vi "Secuencia_Leds.vi"() -> ()   [LabVIEW 2020]
panel:
  out "Array":bool[](array[boolean])
  out "data":bool[](array[boolean])
  out "Numeric":dbl
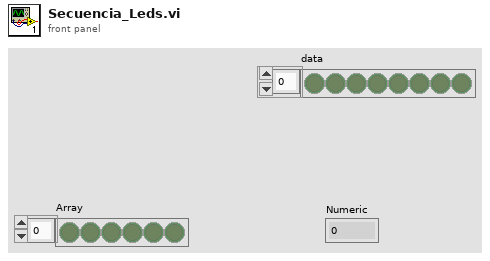
[diagram p1: front panel]
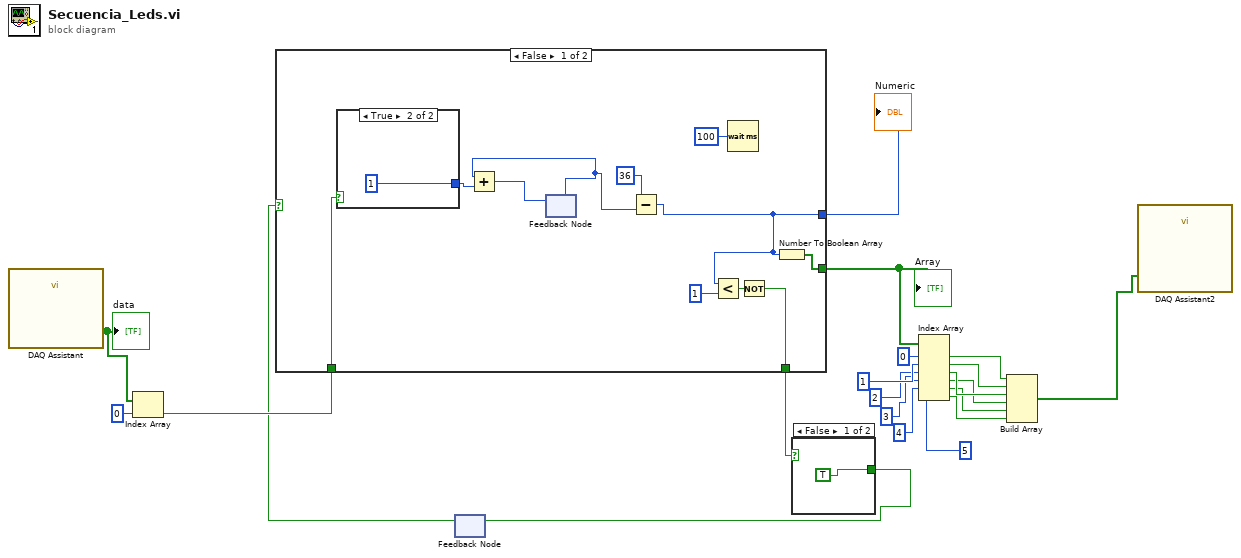
[diagram p0: block diagram]
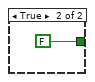
[diagram p2: hidden frame]
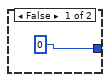
[diagram p3: hidden frame]
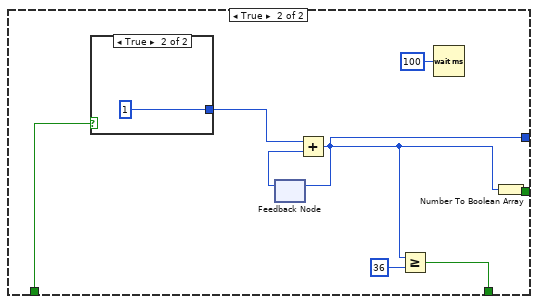
[diagram p4: hidden frame]
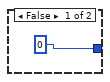
[diagram p5: hidden frame]
diagram:
  n1 = call "DAQ Assistant"() -> ("data"=w21:bool[])  [unwired: 17 in, 2 out]
  "data" <- w21
  n2 = Index Array(array=w21, index=0) -> (element=w19:bool)
  n3 = feedback #1() -> (w2:bool)  [unwired: 1 in]
  n4 = case shown="False" w2 {
    tunnel: [w32 w42] -> w17
    tunnel: w19 -> [w30 w41]
    tunnel: [w25 w37] -> w18
    tunnel: [w23 w35] -> w1
    frame False {
      n5 = case shown="True" w30 {
        tunnel: [0 1] -> w28
        frame False {
        }
        frame True {
        }
      }
      n6 = feedback #2() -> (w27:i32)  [unwired: 1 in]
      n7 = Add(x=w27, y=w28) -> (x+y=w29:i32)
      n8 = feedback-in #2(w29) -> ()
      n9 = Subtract(x=36, y=w27) -> (x-y=w25:i32)
      n10 = Less?(x=w25, y=1) -> (x < y?=w22:bool)
      n11 = Wait (ms)(milliseconds to wait=u32 100) -> ()  [unwired: 1 out]
      n12 = Not(x=w22) -> (.not. x?=w23:bool)
      n13 = Number To Boolean Array(number=w25) -> (Boolean array=w32:bool[])
    }
    frame True {
      n14 = case shown="True" w41 {
        tunnel: [0 1] -> w40
        frame False {
        }
        frame True {
        }
      }
      n15 = feedback #3() -> (w39:i32)  [unwired: 1 in]
      n16 = Add(x=w40, y=w39) -> (x+y=w37:i32)
      n17 = feedback-in #3(w37) -> ()
      n18 = Greater Or Equal?(x=w37, y=36) -> (x >= y?=w35:bool)
      n19 = Wait (ms)(milliseconds to wait=u32 100) -> ()  [unwired: 1 out]
      n20 = Number To Boolean Array(number=w37) -> (Boolean array=w42:bool[])
    }
  }
  "Numeric" <- w18
  "Array" <- w17
  n21 = case shown="False" w1 {
    tunnel: [TRUE FALSE] -> w3
    frame False {
    }
    frame True {
    }
  }
  n22 = feedback-in #1(w3) -> ()
  n23 = Index Array(array=w17, index #1=0 ("index"), index #2=1, index #3=2, index #4=3, index #5=4, index #6=5) -> (element #1=w9:bool, element #2=w8:bool, element #3=w7:bool, element #4=w6:bool, element #5=w5:bool, element #6=w4:bool)
  n24 = Build Array(w9, w8, w7, w6, w5, w4) -> (w10:bool[])
  n25 = call "DAQ Assistant2"("data"=w10) -> ()  [unwired: 17 in, 2 out]
